vi "Step 2 - Perform Decimation Filtering (MRate).vi"() -> ()   [LabVIEW 2023]
doc: "Demonstrates how to use the DFD MRate Filtering VI to perform multirate filtering. In this example, the DFD MRate Filtering VI uses a decimation filter you designed to process a signal that the Multitone Generator VI generates. The DFD MRate Filtering VI then returns both the original signal and the filtered signal.\n\nComplete the following steps to use this VI.\n1) Run the VI.\n2) Examine the Signals graph to observe the effect of decimation filtering.\n3) Examine the block diagram to learn how to use the DFD MRate Filtering VI."
uses:
  <vilib>/addons/Digital Filter Design/Multirate.llb/DFD MRate Filtering (Wfm).vi
  <vilib>/measure/NI_MAPro.lvlib
  <vilib>/addons/Digital Filter Design/NI_DigFilterLicensed.lvlib
panel:
  out "Sampling Frequency of Signal Out [Hz]":dbl
  out "Sampling Frequency of Signal In [Hz]":dbl
  out "Signals":waveform(dbl)[](graph)
  # "Select Help>>Show Context Help and move the cursor over the VI icon for more information."
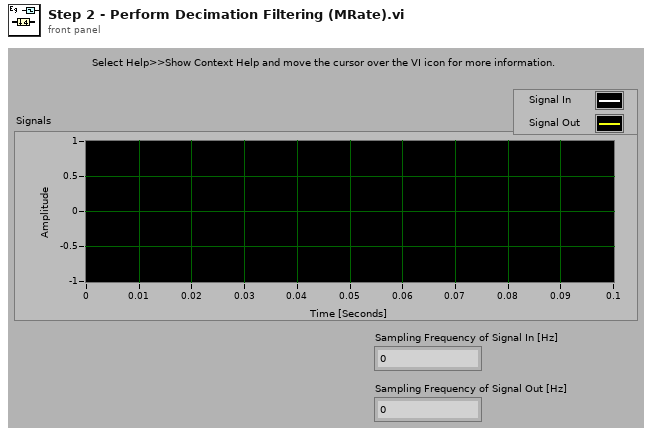
[diagram p1: front panel]
types:
  T1 = typedef "NI_DigFilterLicensed.lvlib/DFD Multirate Filter Obj.ctl" = cluster{"mMRate_Structure":enum16{"CIC", "FIR", "IIR", "Lattice"}, "mMRate_Mode":T2, "mMRate_Factor":i32, "mMRate_FIRParams":cluster{"mMRate_FIR_H":dbl[], "mMRate_FIR_IsNyquist?":bool, "mMRate_FIR_IsSymmetric?":bool}, "mMRate_CICParams":cluster{"mMRate_CIC_#Stage":i32, "mMRate_CIC_Lag":i32, "mMRate_CIC_Type":enum16{"Lowpass", "Highpass"}}, "mMRate_Order":i32, "mMRate_Version":string, "mMRate_Comments":string, "mMRate_RationalFactor":cluster{"mMRate_L":i32, "mMRate_M":i32}, "mMRate_Fs":dbl, "mMRate_Quantized?":bool, "mMRate_QFilterGain":dbl, "mMRate_CoefWl":i16, "mMRate_Scaling":cluster{"mMRate_ScaleByPowerOf2?":bool, "mMRate_ScaleType":T3}, "mMRate_InputWl":i16, "mMRate_OutputWl":i16, "mMRate_OutputMode":T4, "mMRate_MultMode":T5, "mMRate_BitPruning":bool, "mMRate_GainWl":i16, "mMRate_OutputFwl":i16, "mMRate_SumIwl":i16, "mMRate_InputIwl ":i16, "mMRate_SumWl":i16, "mMRate_CoefIwl":i16}
  T2 = typedef "NI_DigFilterLicensed.lvlib/DFD Multirate Mode.ctl" = i16
  T3 = typedef "NI_DigFilterLicensed.lvlib/DFD Coef Norm Type.ctl" = enum16{"No Norm", "Time Domain 1-Norm", "Time Domain 2-Norm", "Time Domain Inf-Norm"}
  T4 = typedef "NI_DigFilterLicensed.lvlib/DFD Round-off Mode.ctl" = enum16{"Nearest", "Truncation"}
  T5 = typedef "NI_DigFilterLicensed.lvlib/DFD FXP MRate Multiply Mode.ctl" = enum16{"Truncated", "Full"}
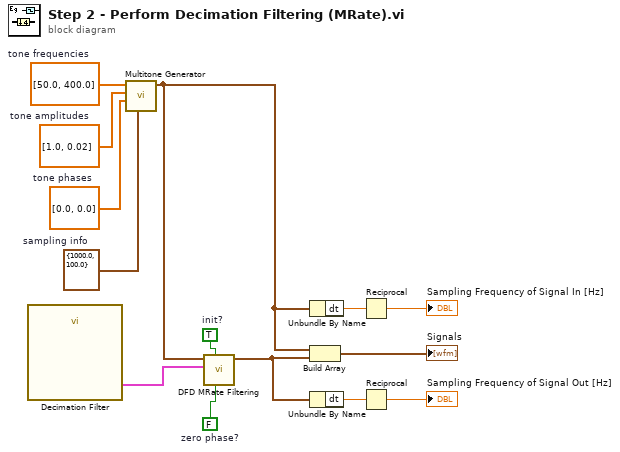
[diagram p0: block diagram]
diagram:
  w11 = dbl[] [0.0, 0.0]  # tone phases
  w12 = FALSE  # zero phase?
  w13 = TRUE  # init?
  w14 = cluster{"Fs":dbl, "#s":dbl} {"Fs"=1000.0, "#s"=100.0}  # sampling info
  w10 = dbl[] [50.0, 400.0]  # tone frequencies
  w2 = dbl[] [1.0, 0.02]  # tone amplitudes
  n1 = call "Decimation Filter"() -> ("multirate filter out"=w1:T1)  [unwired: 11 out]
  n2 = call <vilib>:"Multitone Generator.vi"("sampling info"=w14, "tone phases"=w11, "tone amplitudes"=w2, "tone frequencies"=w10) -> ("signal out"=w8:waveform(dbl))  [unwired: 4 in, 3 out]
  n3 = call-poly <vilib>:"DFD MRate Filtering.vi"("zero phase? (T)"=w12, "init? (F)"=w13, "multirate filter"=w1, "signal in"=w8) -> ("signal out"=w3:waveform(dbl))  [unwired: 1 in, 6 out]
  n4 = Unbundle By Name ("Get Waveform Components")(w8) -> ("dt"=w7:dbl)
  n5 = Build Array(w8, w3) -> (→"Signals":waveform(dbl)[])
  n6 = Unbundle By Name ("Get Waveform Components")(w3) -> ("dt"=w4:dbl)
  n7 = Reciprocal(x=w7) -> (1/x=→"Sampling Frequency of Signal In [Hz]":dbl)
  n8 = Reciprocal(x=w4) -> (1/x=→"Sampling Frequency of Signal Out [Hz]":dbl)
